vi "Find Node.vi"(7 "Node To Index Lookup Map":map{i16, i16[]}(c390), 10 "ID":i32, 11 "Tree":T1[](array[typedef])) -> (2 "Index":i16, 3 "Node":T1={"Node Type"=enum."Path", "ID"=0, "Path Data"={"Path Name"="", "Outcome Name"=""}, "Single Cmd Info"={"Name"="", "CPTM.DataType"=variant, "All Control Values Variant"=[], "icon full"={"image type"=0, "image depth"=0, "image"=[], "mask"=[], "colors"=[], "Rectangle"={"left"=0, "top"=0, "right"=0, "bottom"=0}}, "icon scaled"={"image type"=0, "image depth"=0, "image"=[], "mask"=[], "colors"=[], "Rectangle"={"left"=0, "top"=0, "right"=0, "bottom"=0}}, "Path"=path "", "Subsystem Color"=16777216}, "Child ID"=[], "Parent ID"=0, "Drawing Info"={"X"=0, "Y"=0, "Width"=0, "Height"=0}})   [LabVIEW 2025]
uses:
  Types/Sequencing Tree Node.ctl
  Types/Single Cmd Info.ctl
  <vilib>/picture/picture.llb/imagedata.ctl
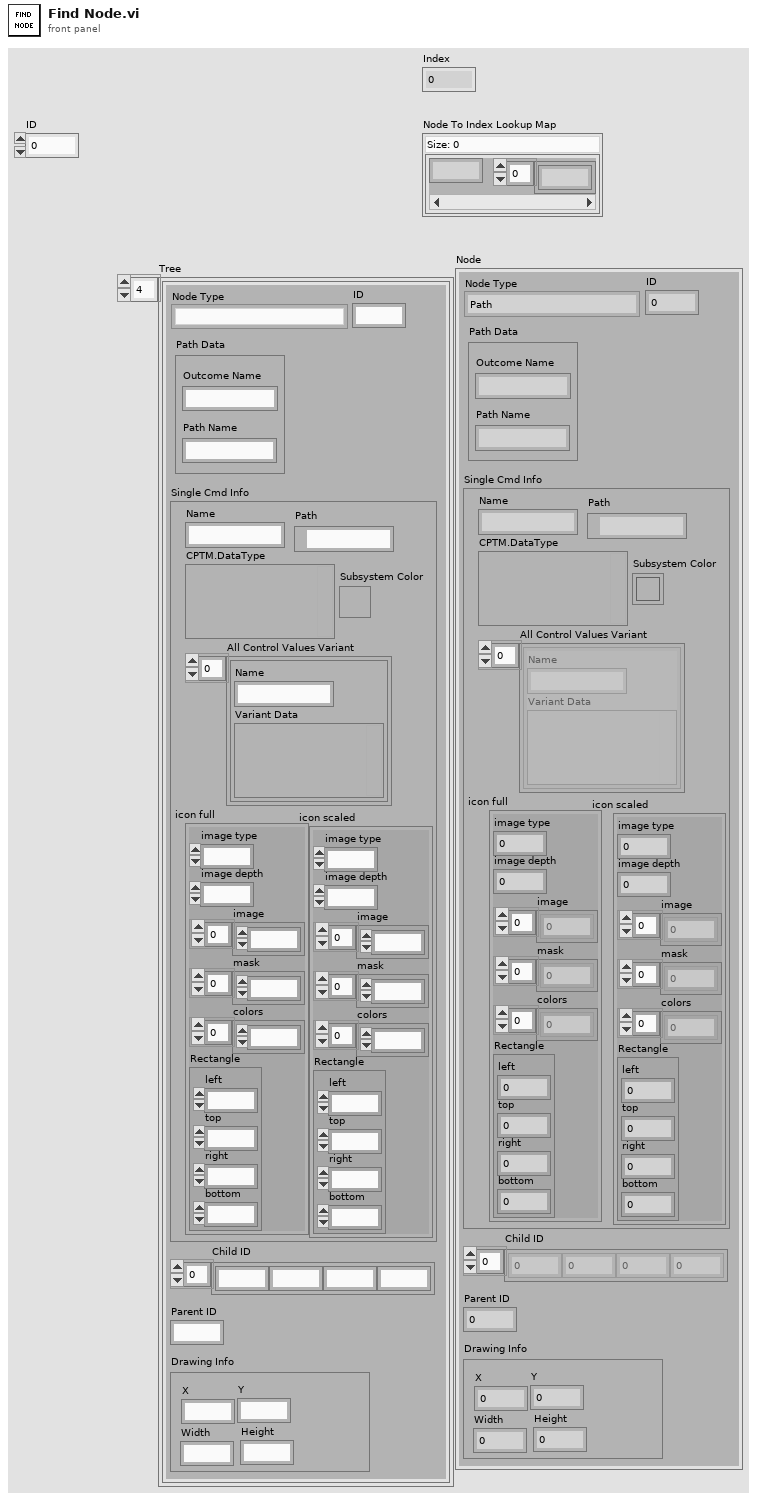
[diagram p1: front panel]
types:
  T1 = typedef "Sequencing Tree Node.ctl" = cluster{"Node Type":enum16{"Path", "Command", "Leaf"}, "ID":i16, "Path Data":cluster{"Path Name":string, "Outcome Name":string}, "Single Cmd Info":T2, "Child ID":i32[], "Parent ID":i32, "Drawing Info":cluster{"X":i32, "Y":i32, "Width":i32, "Height":i32}}
  T2 = typedef "Single Cmd Info.ctl" = cluster{"Name":string, "CPTM.DataType":variant, "All Control Values Variant":cluster{"Name":string, "Variant Data":variant}[], "icon full":T3, "icon scaled":T3, "Path":path, "Subsystem Color":u32}
  T3 = typedef "imagedata.ctl" = cluster{"image type":i32, "image depth":i32, "image":u8[], "mask":u8[], "colors":u32[], "Rectangle":cluster{"left":i16, "top":i16, "right":i16, "bottom":i16}}
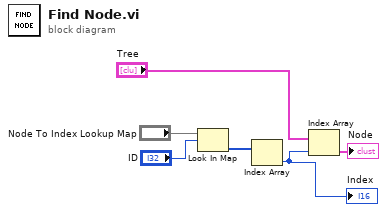
[diagram p0: block diagram]
diagram:
  n1 = Look In Map(map="Node To Index Lookup Map", key="ID") -> (value=w4:i16[])  [unwired: 1 in, 1 out]
  n2 = Index Array(array=w4) -> (element=w1:i16)  [unwired: 1 in]
  "Index" <- w1
  n3 = Index Array(array="Tree", index=w1) -> (element=→"Node":T1)
